vi "Add Error.vi"(8 "error in (no error)":errorcluster, 9 "String to Append":string, 10 "Error":T1, 11 "Insert Error":bool=TRUE) -> (0 "error out":errorcluster)   [LabVIEW 2021, in "CIFCoreCommon.lvlib"]
uses:
  CIFCoreCommon.lvlib
  Typedef/Errors.ctl
  <vilib>/CIF Foundation/CIF Utilities/Errors/Errors_CIF_U.lvlib
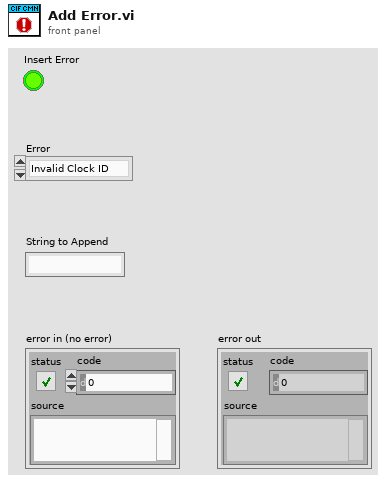
[diagram p1: front panel]
types:
  T1 = typedef "CIFCoreCommon.lvlib/Errors.ctl" = enum16{"Invalid Clock ID", "Long Sleep", "gRPC Server Not Found", "Config Parse", "Timestamp Wrap", "Delayed Execution", "Duplicate Channel", "Missing Channel", "Incorrect Type", "Flatten Error", "Unflatten Data", "Unique Name", "Plugin Not Found", "Plugin Type Not Found", "Plugin Version Not Found", "Manager Not Found", "Numerical Issue", "Time Jump", "Clock ID Match", "Channel Length", "Plugin Connection", "gRPC Server Connection", "PPL Name Match", "Build", "Config Log Parse", "Plugin Load", "UI Subpanel Load", "Python Name", "Invalid Name", "Unable to Change Ch Buffer", "Failed Kill", "Failed SysExec", "Function Not Implemented", "Load Timeout", "Invalid FTE", "Manager Crash"}
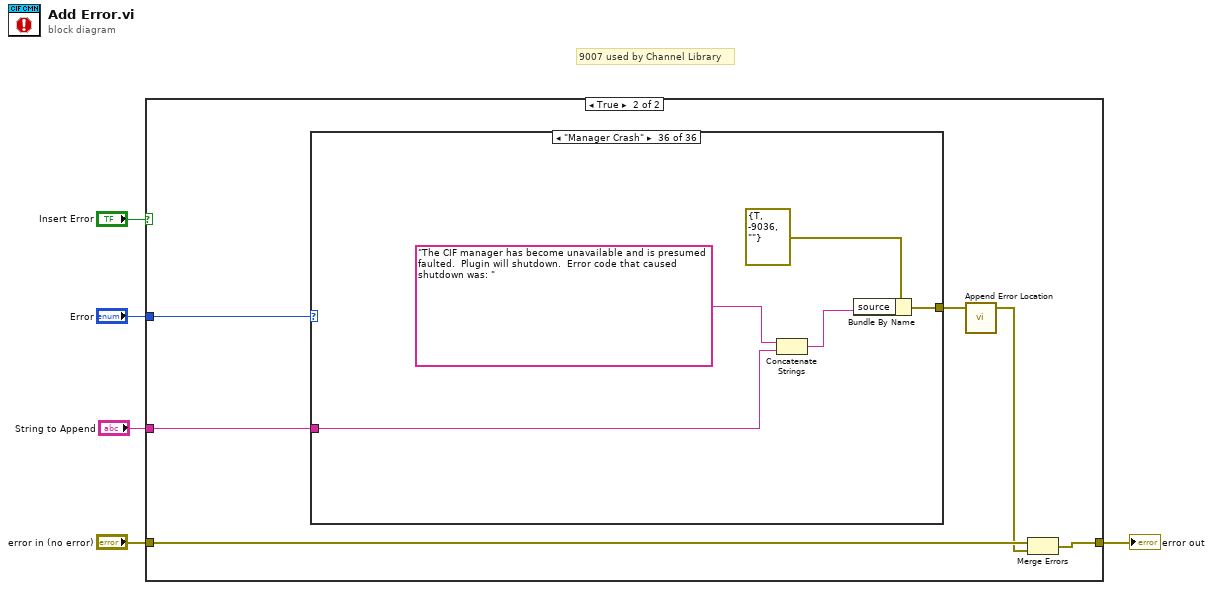
[diagram p0: block diagram]
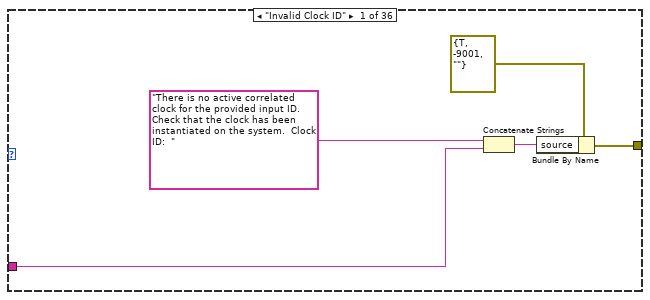
[diagram p3: hidden frame]
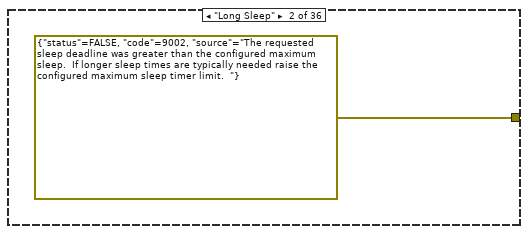
[diagram p4: hidden frame]
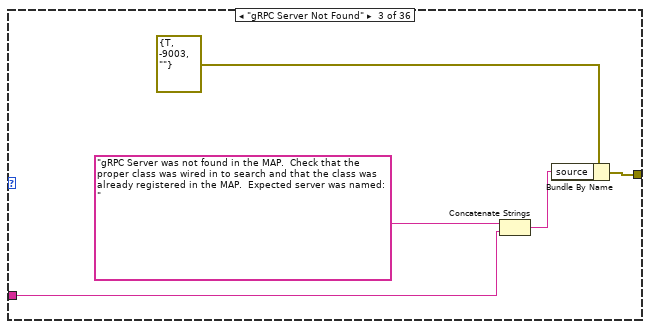
[diagram p5: hidden frame]
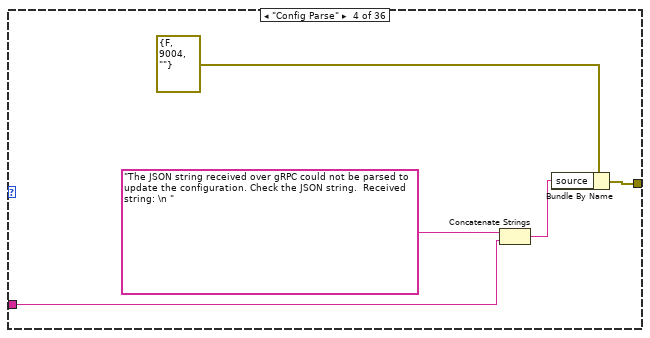
[diagram p6: hidden frame]
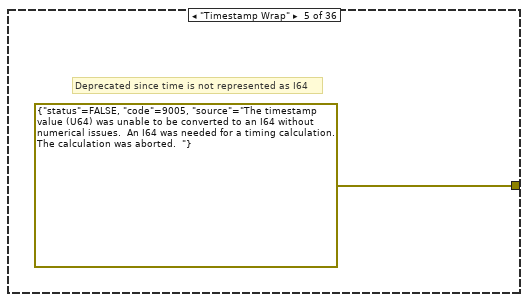
[diagram p7: hidden frame]
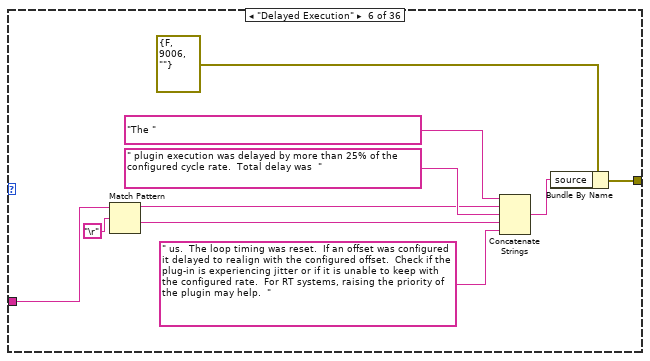
[diagram p8: hidden frame]
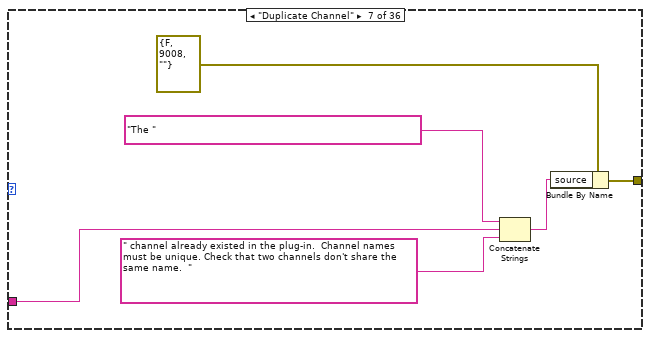
[diagram p9: hidden frame]
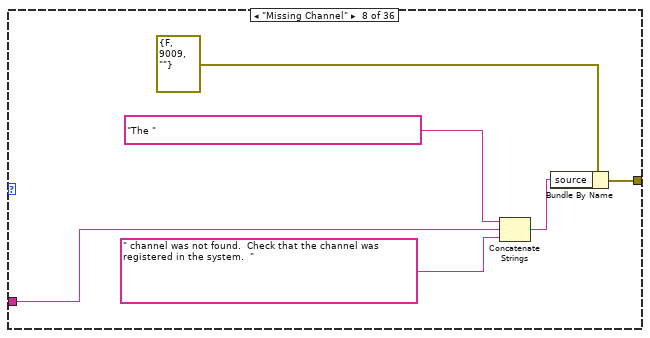
[diagram p10: hidden frame]
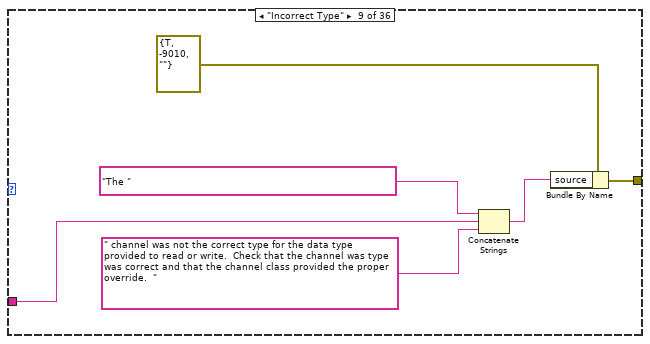
[diagram p11: hidden frame]
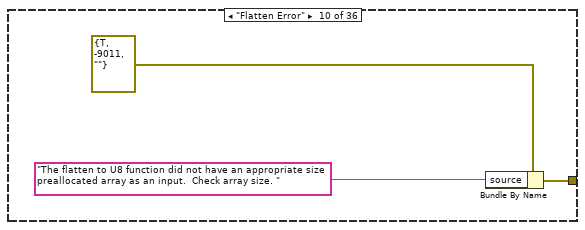
[diagram p12: hidden frame]
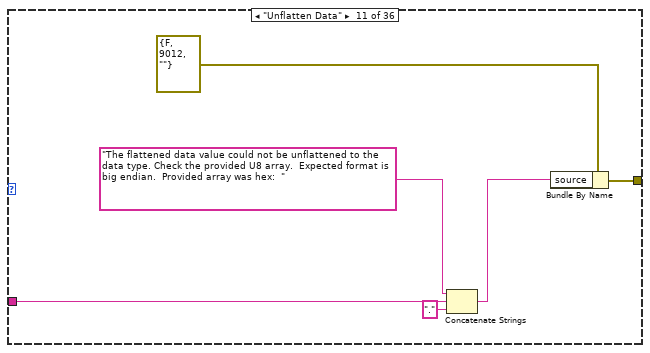
[diagram p13: hidden frame]
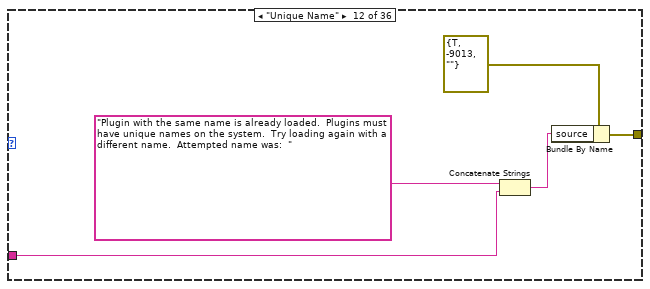
[diagram p14: hidden frame]
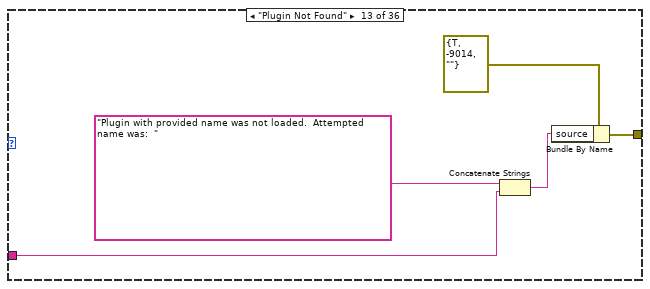
[diagram p15: hidden frame]
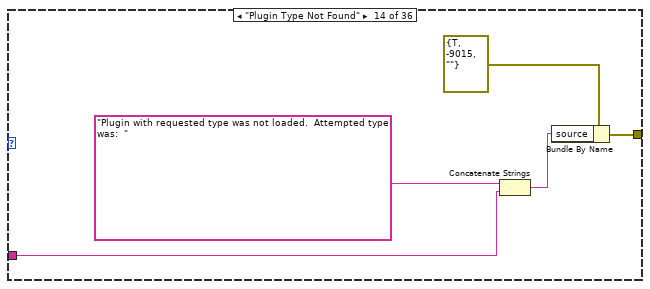
[diagram p16: hidden frame]
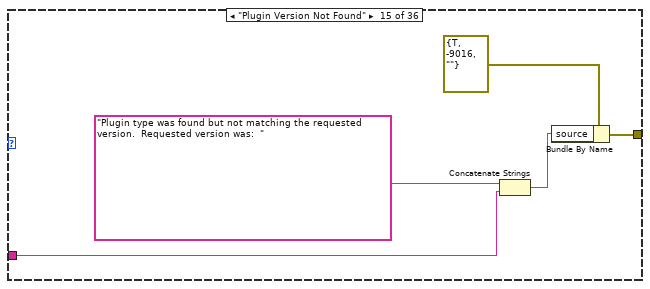
[diagram p17: hidden frame]
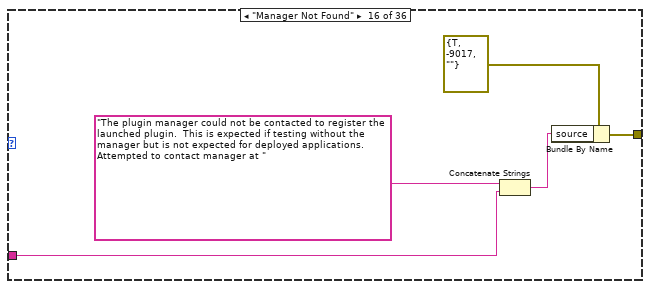
[diagram p18: hidden frame]
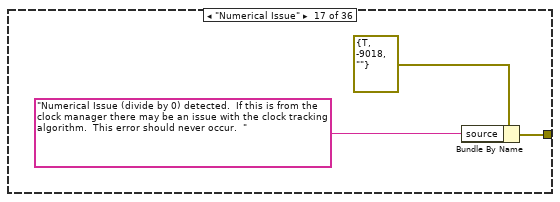
[diagram p19: hidden frame]
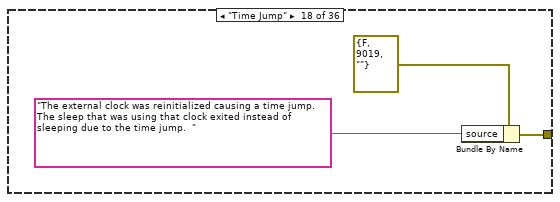
[diagram p20: hidden frame]
diagram:
  # "9007 used by Channel Library"
  n1 = case shown="True" "Insert Error" {
    tunnel: [w6 w9] -> w4
    tunnel: "error in (no error)" -> [w6 w10]
    tunnel: "Error" -> [_ w12]
    tunnel: "String to Append" -> [_ w11]
    frame False {
    }
    frame True {
      n2 = case shown="\"Manager Crash\"" w12 {
        tunnel: w11 -> [w14 _ w20 w25 _ w34 w42 w46 w52 _ w63 w68 w73 w78 w83 w88 _ _ _ _ w104 w109 w114 w119 w124 _ _ w135 w140 _ w149 w154 w159 w164 w169 w173]
        tunnel: [w16 errorcluster {"status"=FALSE, "code"=9002, "source"="The requested sleep deadline was greater than the configured maximum sleep.  If longer sleep times are typically needed raise the configured maximum sleep timer limit.  "} ("Invalid ID") w22 w27 errorcluster {"status"=FALSE, "code"=9005, "source"="The timestamp value (U64) was unable to be converted to an I64 without numerical issues.  An I64 was needed for a timing calculation.  The calculation was aborted.  "} ("Invalid ID") w38 w44 w50 w56 w59 w65 w70 w75 w80 w85 w90 w93 w96 w99 w102 w107 w112 w117 w122 w127 w130 w133 w138 w143 w146 w151 w156 w161 w166 w171 w176] -> w8
        frame "Invalid Clock ID" {
          n3 = Concatenate Strings("There is no active correlated clock for the provided input ID.  Check that the clock has been instantiated on the system.  Clock ID:  " ("source"), w14) -> (w13:string)
          n4 = Bundle By Name(cluster=errorcluster {"status"=TRUE, "code"=-9001, "source"=""} ("Invalid ID"), "source"=w13) -> (w16:errorcluster)
        }
        frame "Long Sleep" {
        }
        frame "gRPC Server Not Found" {
          n5 = Concatenate Strings("gRPC Server was not found in the MAP.  Check that the proper class was wired in to search and that the class was already registered in the MAP.  Expected server was named:  " ("source"), w20) -> (w21:string)
          n6 = Bundle By Name(cluster=errorcluster {"status"=TRUE, "code"=-9003, "source"=""} ("Invalid ID"), "source"=w21) -> (w22:errorcluster)
        }
        frame "Config Parse" {
          n7 = Concatenate Strings("The JSON string received over gRPC could not be parsed to update the configuration. Check the JSON string.  Received string: \n " ("source"), w25) -> (w26:string)
          n8 = Bundle By Name(cluster=errorcluster {"status"=FALSE, "code"=9004, "source"=""} ("Invalid ID"), "source"=w26) -> (w27:errorcluster)
        }
        frame "Timestamp Wrap" {
          # "Deprecated since time is not represented as I64"
        }
        frame "Delayed Execution" {
          n9 = Match Pattern(string=w34, regular expression="\r") -> (before substring=w33:string, after substring=w31:string)  [unwired: 1 in, 2 out]
          n10 = Concatenate Strings("The " ("source"), w33, " plugin execution was delayed by more than 25% of the configured cycle rate.  Total delay was  " ("source"), w31, " us.  The loop timing was reset.  If an offset was configured it delayed to realign with the configured offset.  Check if the plug-in is experiencing jitter or if it is unable to keep with the configured rate.  For RT systems, raising the priority of the plugin may help.  " ("source")) -> (w37:string)
          n11 = Bundle By Name(cluster=errorcluster {"status"=FALSE, "code"=9006, "source"=""} ("Invalid ID"), "source"=w37) -> (w38:errorcluster)
        }
        frame "Duplicate Channel" {
          n12 = Concatenate Strings("The " ("source"), w42, " channel already existed in the plug-in.  Channel names must be unique. Check that two channels don't share the same name.  " ("source")) -> (w43:string)
          n13 = Bundle By Name(cluster=errorcluster {"status"=FALSE, "code"=9008, "source"=""} ("Invalid ID"), "source"=w43) -> (w44:errorcluster)
        }
        frame "Missing Channel" {
          n14 = Concatenate Strings("The " ("source"), w46, " channel was not found.  Check that the channel was registered in the system.  " ("source")) -> (w49:string)
          n15 = Bundle By Name(cluster=errorcluster {"status"=FALSE, "code"=9009, "source"=""} ("Invalid ID"), "source"=w49) -> (w50:errorcluster)
        }
        frame "Incorrect Type" {
          n16 = Concatenate Strings("The " ("source"), w52, " channel was not the correct type for the data type provided to read or write.  Check that the channel was type was correct and that the channel class provided the proper override.  " ("source")) -> (w53:string)
          n17 = Bundle By Name(cluster=errorcluster {"status"=TRUE, "code"=-9010, "source"=""} ("Invalid ID"), "source"=w53) -> (w56:errorcluster)
        }
        frame "Flatten Error" {
          n18 = Bundle By Name(cluster=errorcluster {"status"=TRUE, "code"=-9011, "source"=""} ("Invalid ID"), "source"="The flatten to U8 function did not have an appropriate size preallocated array as an input.  Check array size. ") -> (w59:errorcluster)
        }
        frame "Unflatten Data" {
          n19 = Concatenate Strings("The flattened data value could not be unflattened to the data type. Check the provided U8 array.  Expected format is big endian.  Provided array was hex:  " ("source"), w63, "." ("string")) -> (w61:string)
          n20 = Bundle By Name(cluster=errorcluster {"status"=FALSE, "code"=9012, "source"=""} ("Invalid ID"), "source"=w61) -> (w65:errorcluster)
        }
        frame "Unique Name" {
          n21 = Concatenate Strings("Plugin with the same name is already loaded.  Plugins must have unique names on the system.  Try loading again with a different name.  Attempted name was:  " ("source"), w68) -> (w69:string)
          n22 = Bundle By Name(cluster=errorcluster {"status"=TRUE, "code"=-9013, "source"=""} ("Invalid ID"), "source"=w69) -> (w70:errorcluster)
        }
        frame "Plugin Not Found" {
          n23 = Concatenate Strings("Plugin with provided name was not loaded.  Attempted name was:  " ("source"), w73) -> (w74:string)
          n24 = Bundle By Name(cluster=errorcluster {"status"=TRUE, "code"=-9014, "source"=""} ("Invalid ID"), "source"=w74) -> (w75:errorcluster)
        }
        frame "Plugin Type Not Found" {
          n25 = Concatenate Strings("Plugin with requested type was not loaded.  Attempted type was:  " ("source"), w78) -> (w79:string)
          n26 = Bundle By Name(cluster=errorcluster {"status"=TRUE, "code"=-9015, "source"=""} ("Invalid ID"), "source"=w79) -> (w80:errorcluster)
        }
        frame "Plugin Version Not Found" {
          n27 = Concatenate Strings("Plugin type was found but not matching the requested version.  Requested version was:  " ("source"), w83) -> (w84:string)
          n28 = Bundle By Name(cluster=errorcluster {"status"=TRUE, "code"=-9016, "source"=""} ("Invalid ID"), "source"=w84) -> (w85:errorcluster)
        }
        frame "Manager Not Found" {
          n29 = Concatenate Strings("The plugin manager could not be contacted to register the launched plugin.  This is expected if testing without the manager but is not expected for deployed applications.  Attempted to contact manager at " ("source"), w88) -> (w89:string)
          n30 = Bundle By Name(cluster=errorcluster {"status"=TRUE, "code"=-9017, "source"=""} ("Invalid ID"), "source"=w89) -> (w90:errorcluster)
        }
        frame "Numerical Issue" {
          n31 = Bundle By Name(cluster=errorcluster {"status"=TRUE, "code"=-9018, "source"=""} ("Invalid ID"), "source"="Numerical Issue (divide by 0) detected.  If this is from the clock manager there may be an issue with the clock tracking algorithm.  This error should never occur.  ") -> (w93:errorcluster)
        }
        frame "Time Jump" {
          n32 = Bundle By Name(cluster=errorcluster {"status"=FALSE, "code"=9019, "source"=""} ("Invalid ID"), "source"="The external clock was reinitialized causing a time jump.  The sleep that was using that clock exited instead of sleeping due to the time jump.  ") -> (w96:errorcluster)
        }
        frame "Clock ID Match" {
          n33 = Bundle By Name(cluster=errorcluster {"status"=FALSE, "code"=9020, "source"=""} ("Invalid ID"), "source"="An update command for an external clock was received but the clock name did not match the exiting clock name.   ") -> (w99:errorcluster)
        }
        frame "Channel Length" {
          n34 = Bundle By Name(cluster=errorcluster {"status"=TRUE, "code"=-9021, "source"=""} ("Invalid ID"), "source"="The internal length of the channel was incorrect.  The length should be set automatically so this is a developer error.  ") -> (w102:errorcluster)
        }
        frame "Plugin Connection" {
          n35 = Concatenate Strings("The plugin could not be found to complete the operation.  The requested plugin was: " ("source"), w104) -> (w105:string)
          n36 = Bundle By Name(cluster=errorcluster {"status"=TRUE, "code"=-9022, "source"=""} ("Invalid ID"), "source"=w105) -> (w107:errorcluster)
        }
        frame "gRPC Server Connection" {
          n37 = Concatenate Strings("The gRPC Server could not be connected.  The attempted address was: " ("source"), w109) -> (w110:string)
          n38 = Bundle By Name(cluster=errorcluster {"status"=TRUE, "code"=-9023, "source"=""} ("Invalid ID"), "source"=w110) -> (w112:errorcluster)
        }
        frame "PPL Name Match" {
          n39 = Concatenate Strings("Build was aborted to fix configuration.  The PPL name did not match the name of the build project or the version of the library did not match.  For UI builds, Instrument Studio requires the name of the PPL match the project.   The name and version were automatically updated.  It should build if you execute the build again.  " ("source"), w114) -> (w115:string)
          n40 = Bundle By Name(cluster=errorcluster {"status"=TRUE, "code"=-9024, "source"=""} ("Invalid ID"), "source"=w115) -> (w117:errorcluster)
        }
        frame "Build" {
          n41 = Concatenate Strings("Build was aborted to due to a parsing error in the pre or post build action.  It may be possible to remove the pre/post-build steps and manually perform pre/post build scripting steps.  " ("source"), w119) -> (w120:string)
          n42 = Bundle By Name(cluster=errorcluster {"status"=TRUE, "code"=-9025, "source"=""} ("Invalid ID"), "source"=w120) -> (w122:errorcluster)
        }
        frame "Config Log Parse" {
          n43 = Concatenate Strings("Config log file could not be parsed to created automated orchestration code.  Issue with line: " ("source"), w124) -> (w125:string)
          n44 = Bundle By Name(cluster=errorcluster {"status"=FALSE, "code"=9026, "source"=""} ("Invalid ID"), "source"=w125) -> (w127:errorcluster)
        }
        frame "Plugin Load" {
          # "Existing error code reused.  Message updated."
          n45 = Bundle By Name(cluster=errorcluster {"status"=TRUE, "code"=1003, "source"=""} ("Invalid ID"), "source"="The built plugin could not be loaded on the system by LabVIEW.  This can be caused by a missing dependency on the system (missing dll/so or called PPL) or by a malleable vi (vim) used on a LabVIEW Class wire (limitation of LabVIEW classes built as PPLs).  Recommended debug steps.  Assure the plugin code will run in interactive/debug mode.  Build sub-sections of the plugin until you can identify the parts that cause built PPLs to not load.  Check for debugging/benchmarking where the \"Get Timestamp.vim\" was used to make sure it is not on a Class wire.   ") -> (w130:errorcluster)
        }
        frame "UI Subpanel Load" {
          n46 = Bundle By Name(cluster=errorcluster {"status"=TRUE, "code"=-9027, "source"=""} ("Invalid ID"), "source"="The UI subpanels could not be loaded on the system.  This is normally due to an incorrect installation.  The subpanels are loaded dynamically from a built PPL.  The subpanel library (CIF Manager UI.x.x.x.lvlibp) is expected at <default CIF directory>\\PluginUI.  On Windows this is C:\\Users\\Public\\Documents\\CIF\\PluginUI.  Recommended debug steps.  Check that the file and directory exist and if needed repair installation.    ") -> (w133:errorcluster)
        }
        frame "Python Name" {
          n47 = Concatenate Strings("The name is not a valid Python variable name.  To facilitate Python orchestration it is recommended to change the name to:  " ("source"), w135) -> (w136:string)
          n48 = Bundle By Name(cluster=errorcluster {"status"=FALSE, "code"=9028, "source"=""} ("Invalid ID"), "source"=w136) -> (w138:errorcluster)
        }
        frame "Invalid Name" {
          n49 = Concatenate Strings("The name is not a valid.  The attempted name was:  " ("source"), w140) -> (w141:string)
          n50 = Bundle By Name(cluster=errorcluster {"status"=TRUE, "code"=-9029, "source"=""} ("Invalid ID"), "source"=w141) -> (w143:errorcluster)
        }
        frame "Unable to Change Ch Buffer" {
          n51 = Bundle By Name(cluster=errorcluster {"status"=FALSE, "code"=9030, "source"=""} ("Invalid ID"), "source"="A request to change the channel buffer size was made but a subscriber is already connected or the plugin is executing so the size cannot be changed.  Buffer size changes must be made when the plugin is not executing and no subcribers are connected to the FIFO channel.  ") -> (w146:errorcluster)
        }
        frame "Failed Kill" {
          n52 = Concatenate Strings("Failed to kill.  The command and response were:" ("source"), w149) -> (w148:string)
          n53 = Bundle By Name(cluster=errorcluster {"status"=FALSE, "code"=9031, "source"=""} ("Invalid ID"), "source"=w148) -> (w151:errorcluster)
        }
        frame "Failed SysExec" {
          n54 = Concatenate Strings("Failed call to sys exec. The command, error, and response were:" ("source"), w154) -> (w153:string)
          n55 = Bundle By Name(cluster=errorcluster {"status"=TRUE, "code"=-9032, "source"=""} ("Invalid ID"), "source"=w153) -> (w156:errorcluster)
        }
        frame "Function Not Implemented" {
          n56 = Concatenate Strings("The requested function has not been implemented.  Requested function was: " ("source"), w159) -> (w158:string)
          n57 = Bundle By Name(cluster=errorcluster {"status"=TRUE, "code"=-9033, "source"=""} ("Invalid ID"), "source"=w158) -> (w161:errorcluster)
        }
        frame "Load Timeout" {
          n58 = Concatenate Strings("The operation to load an external component timed out.  Component and requestor details were: " ("source"), w164) -> (w163:string)
          n59 = Bundle By Name(cluster=errorcluster {"status"=TRUE, "code"=-9034, "source"=""} ("Invalid ID"), "source"=w163) -> (w166:errorcluster)
        }
        frame "Invalid FTE" {
          n60 = Concatenate Strings("The future time event provided was out of range.  The provided FTE and system time were: " ("source"), w169) -> (w168:string)
          n61 = Bundle By Name(cluster=errorcluster {"status"=FALSE, "code"=9035, "source"=""} ("Invalid ID"), "source"=w168) -> (w171:errorcluster)
        }
        frame "Manager Crash" {
          n62 = Concatenate Strings("The CIF manager has become unavailable and is presumed faulted.  Plugin will shutdown.  Error code that caused shutdown was: " ("source"), w173) -> (w174:string)
          n63 = Bundle By Name(cluster=errorcluster {"status"=TRUE, "code"=-9036, "source"=""} ("Invalid ID"), "source"=w174) -> (w176:errorcluster)
        }
      }
      n64 = call <vilib>:"Append Error Location.vi"("error in (no error)"=w8) -> ("error out"=w7:errorcluster)  [unwired: 4 in]
      n65 = Merge Errors(w10, w7) -> (w9:errorcluster)
    }
  }
  "error out" <- w4
